vi "Unpack for gRPC.vi"(8 "error in":errorcluster, 9 "configuration / results":enum16{"Configuration", "Results"}(ring), 10 "any":T1, 11 "measurement customizations in":refnum<class "Measurement Plugin.lvclass">) -> (0 "error out":errorcluster, 2 "data value":variant, 3 "measurement customizations out":refnum<class "Measurement Plugin.lvclass">)   [LabVIEW 2021, in "channelGanging.lvlib" / "Measurement Plugin.lvclass"]
uses:
  Measurement Plugin.lvclass
  Measurement Plugin.lvclass/Measurement Plugin.ctl
  Measurement Configuration.ctl
  channelGanging.lvlib
  Measurement Results.ctl
  3ecd018e-d556-4cbc-bc60-c4ba57204520.vi
  a521b266-ce99-437c-923d-067dcf1e07fd.vi
  <vilib>/MeasurementLink/MeasurementLink Measurement Server/Measurement Plugin Service/Measurement Plugin Service.lvclass
  C:/Program Files/National Instruments/LabVIEW 2021/vi.lib/MeasurementLink/MeasurementLink Measurement Server/Measurement Plugin Service/Measurement Plugin Service.lvclass
  C:/Users/Administrator/Documents/GitHub/pmic-labview/source/measurements/channelGanging/channelGanging/Advanced/Measurement Plugin.lvclass
  <vilib>/gRPC/LabVIEW gRPC Library/Shared/Any.ctl
  <vilib>/gRPC/LabVIEW gRPC Library/grpc-lvsupport-release.lvlib
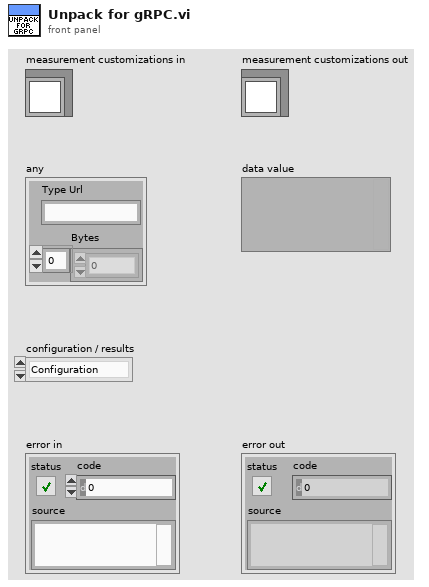
[diagram p1: front panel]
types:
  T1 = typedef "grpc-lvsupport-release.lvlib/Any.ctl" = cluster{"Type Url":string, "Bytes":u8[]}
  T2 = typedef "grpc-lvsupport-release.lvlib/grpcId.ctl" = u64
  T3 = typedef "channelGanging.lvlib/Measurement Configuration.ctl" = cluster{"Source input channels":i32[], "Source resource names":string[], "Source channel mode":enum32{"Master", "Slave", "Slave- inverted"}[], "Source system configuration":enum16{"Parallel", "Series"}, "Source voltage level":dbl, "Source voltage level range":dbl, "Source sense":enum16{"Remote", "Local"}, "Source limit symmetry":enum16{"Asymmetric", "Symmetric"}, "Source current limit range":dbl, "Source current limit low":dbl, "Source current limit high":dbl, "Source aperture time":dbl, "Source transient response":enum16{"Fast", "Normal", "Slow"}, "Load input channels":i32[], "Load resource names":string[], "Load channel mode":enum32{"Master", "Slave", "Slave- inverted"}[], "Load system configuration":enum16{"Parallel", "Series"}, "Load current Level":dbl, "Load current level range":dbl, "Load Sense":enum16{"Remote", "Local"}, "Load limit symmetry":enum16{"Asymmetric", "Symmetric"}, "Load voltage limit range":dbl, "Load voltage limit low":dbl, "Load voltage limit high":dbl, "Load aperture time":dbl, "Load transient response":enum16{"Fast", "Normal", "Slow"}, "Measurement time":dbl}
  T4 = typedef "channelGanging.lvlib/Measurement Results.ctl" = cluster{"dt 2":dbl, "Source voltages":dbl[], "Source currents":dbl[], "Load voltages":dbl[], "Load currents":dbl[]}
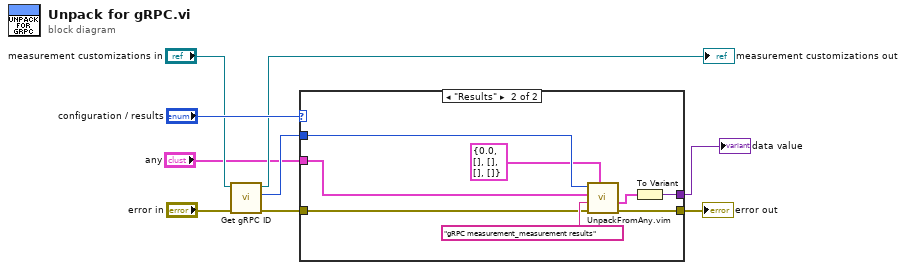
[diagram p0: block diagram]
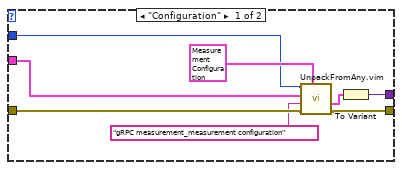
[diagram p2: hidden frame]
diagram:
  n1 = call <vilib>:"Get gRPC ID.vi"("error in"="error in", "measurement plugin service in"="measurement customizations in") -> ("error out"=w6:errorcluster, "gRPC ID"=w3:T2, "measurement plugin service out"=→"measurement customizations out":refnum<class "Measurement Plugin.lvclass">)  [unwired: 7 in]
  n2 = case shown="\"Results\"" "configuration / results" {
    tunnel: w6 -> [w15 w19]
    tunnel: "any" -> [w10 w18]
    tunnel: w3 -> [w12 w22]
    tunnel: [w16 w23] -> w9
    tunnel: [w17 w25] -> w1
    frame "Configuration" {
      n3 = call "UnpackFromAny.vim"("Data Type"=T3 {"Source input channels"=[], "Source resource names"=[], "Source channel mode"=[], "Source system configuration"=enum."Parallel", "Source voltage level"=2.0, "Source voltage level range"=20.0, "Source sense"=enum."Remote", "Source limit symmetry"=enum."Asymmetric", "Source current limit range"=2.0, "Source current limit low"=2.0, "Source current limit high"=20.0, "Source aperture time"=0.01, "Source transient response"=enum."Slow", "Load input channels"=[], "Load resource names"=[], "Load channel mode"=[], "Load system configuration"=enum."Parallel", "Load current Level"=2.0, "Load current level range"=20.0, "Load Sense"=enum."Remote", "Load limit symmetry"=enum."Asymmetric", "Load voltage limit range"=2.0, "Load voltage limit low"=2.0, "Load voltage limit high"=20.0, "Load aperture time"=0.01, "Load transient response"=enum."Slow", "Measurement time"=0.01} ("Measurement Configuration"), "error in"=w15, "Message Type"="gRPC measurement_measurement configuration", "Any"=w10, "gRPCid in"=w12) -> ("error out"=w16:errorcluster, "Unpacked Value"=w14:T3)  [unwired: 4 in, 1 out]
      n4 = To Variant(anything=w14) -> (Variant=w17:variant)
    }
    frame "Results" {
      n5 = call "UnpackFromAny.vim"("Data Type"=T4 {"dt 2"=0.0, "Source voltages"=[], "Source currents"=[], "Load voltages"=[], "Load currents"=[]} ("Measurement Results"), "error in"=w19, "Message Type"="gRPC measurement_measurement results", "Any"=w18, "gRPCid in"=w22) -> ("error out"=w23:errorcluster, "Unpacked Value"=w24:T4)  [unwired: 4 in, 1 out]
      n6 = To Variant(anything=w24) -> (Variant=w25:variant)
    }
  }
  "error out" <- w9
  "data value" <- w1
